vi "Event Handler.vi"(8 "error in (no error)":errorcluster, 10 "Stop Event Handler":refnum<user-event>, 11 "DataGrid in":refnum<class "DataGrid.lvclass">) -> (0 "error out":errorcluster)   [LabVIEW 2017, in "DataGrid.lvclass"]
doc: "The <b>Event Handler VI</b> is a dynamic dispatch VI that should be overwritten if events are needed to create the enhanced QControl. \n\nBy inheriting from the main Control.lvclass the overwritten <b>Event Handler VI</b> will be launched asynchronously in the initialization of the QControl.\n<b> </b> <b> </b>\n©2016 Q Software Innovations, LLC (QSI)\nwritten by Quentin Alldredge\nproduced in LabVIEW 2015\n\nsupport@qsoftwareinnovations.com\nwww.qsoftwareinnovations.com\n\nAll rights reserved.\n\nRedistribution and use in source and binary forms, with or without modification, are permitted provided that the following conditions are met:\n\n * Redistributions of source code must retain the above copyright notice, this list of conditions and the following disclaimer.\n * Redistributions in binary form must reproduce the above copyright notice, this list of conditions and the following disclaimer in the documentation and/or other materials provided with the distribution.\n * Neither the name of Q Software Innovations, LLC. nor the names of its contributors may be used to endorse or promote products derived from this software without specific prior written permission.\n\nTHIS SOFTWARE IS PROVIDED BY THE COPYRIGHT HOLDERS AND CONTRIBUTORS \"AS IS\" AND ANY EXPRESS OR IMPLIED WARRANTIES, INCLUDING, BUT NOT LIMITED TO, THE IMPLIED WARRANTIES OF MERCHANTABILITY AND FITNESS FOR A PARTICULAR PURPOSE ARE DISCLAIMED. IN NO EVENT SHALL THE COPYRIGHT OWNER OR CONTRIBUTORS BE LIABLE FOR ANY DIRECT, INDIRECT, INCIDENTAL, SPECIAL, EXEMPLARY, OR CONSEQUENTIAL DAMAGES (INCLUDING, BUT NOT LIMITED TO, PROCUREMENT OF SUBSTITUTE GOODS OR SERVICES; LOSS OF USE, DATA, OR PROFITS; OR BUSINESS INTERRUPTION) HOWEVER CAUSED AND ON ANY THEORY OF LIABILITY, WHETHER IN CONTRACT, STRICT LIABILITY, OR TORT (INCLUDING NEGLIGENCE OR OTHERWISE) ARISING IN ANY WAY OUT OF THE USE OF THIS SOFTWARE, EVEN IF ADVISED OF THE POSSIBILITY OF SUCH DAMAGE."
uses:
  DataGrid.lvclass
  DataGrid.lvclass/DataGrid.ctl
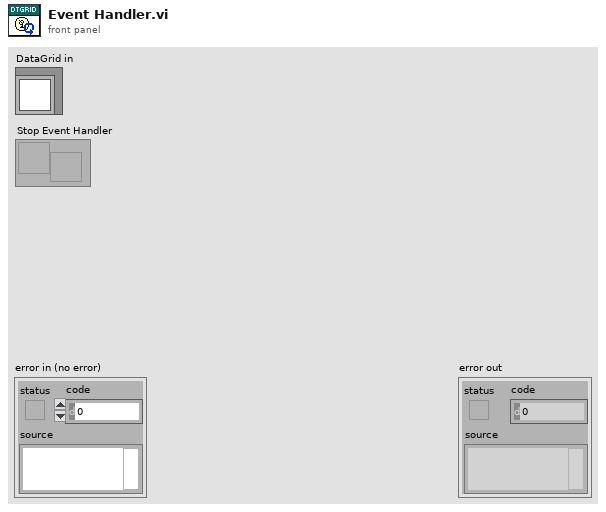
[diagram p1: front panel]
types:
  T1 = typedef "LVPoint32TypeDef.ctl" = cluster{"Horizontal":i32, "Vertical":i32}
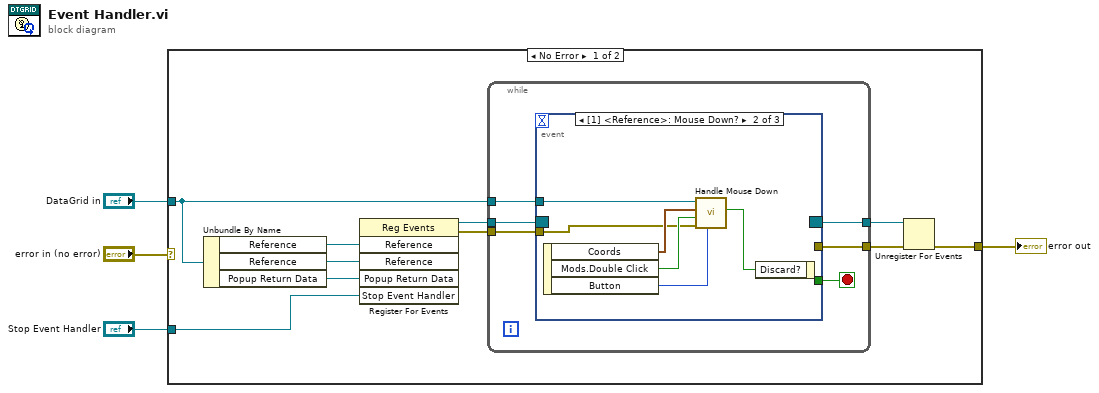
[diagram p0: block diagram]
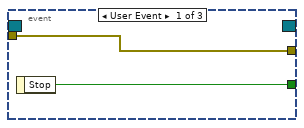
[diagram p2: hidden frame]
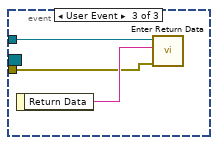
[diagram p3: hidden frame]
diagram:
  n1 = case shown="No Error" "error in (no error)" {
    selector: "error in (no error)" -> [_ w32]
    tunnel: [w11 w32] -> w3
    tunnel: "DataGrid in" -> [w9 _]
    tunnel: "Stop Event Handler" -> [w7 _]
    frame No Error {
      n2 = Unbundle By Name(w9) -> ("Reference"=w8:refnum<vi>, "Reference"=w5:refnum<vi>, "Popup Return Data"=w6:refnum<user-event>)
      n3 = register-events(w8, w5, w6, w7) -> (reference out=w14:refnum<event-registration>, error out=w13:errorcluster)  [unwired: 2 in]
      n4 = while {
        tunnel: w14 -> [w20]
        tunnel: w13 -> [w18]
        tunnel: [w17] -> w12
        tunnel: [w15] -> w10
        tunnel: w9 -> [w19]
        stop <- w16 stop-if-true
        n5 = event shown="[1] <Reference>: Mouse Down?" {
          selector: w20 -> [_ _ _]
          dyn-events: [_ _ _] -> w15
          timeout: _ -> [_ _ _]
          tunnel: w19 -> [_ w28 w31]
          tunnel: w18 -> [w22 w24 w29]
          tunnel: [w22 _ _] -> w17
          tunnel: [w21 _ _] -> w16
          event User Event {
            n6 = event-data() -> ("Stop"=w21:bool)  [unwired: 1 in]
          }
          event Mouse Down? {
            n7 = event-data() -> ("Coords"=w27:T1, "Mods.Double Click"=w26:bool, "Button"=w23:u16)  [unwired: 1 in]
            n8 = call "Handle Mouse Down.vi"("Button"=w23, "error in (no error)"=w24, "Double Click"=w26, "Coords"=w27, "DataGrid in"=w28) -> ("Discard?"=w25:bool)  [unwired: 4 in, 2 out]
            n9 = event-data("Discard?"=w25) -> ()  [unwired: 1 in, 1 out]
          }
          event User Event {
            n10 = event-data() -> ("Return Data"=w30:string)  [unwired: 1 in]
            n11 = call "Enter Return Data.vi"("error in (no error)"=w29, "Return Data"=w30, "DataGrid in"=w31) -> ()  [unwired: 7 in, 2 out]
          }
        }
      }
      n12 = Unregister For Events(event registration refnum=w10, error in=w12) -> (error out=w11:errorcluster)
    }
    frame Error {
    }
  }
  "error out" <- w3
